vi "source_measure.vi"(8 "error in (no error)":errorcluster, 11 "Input parameters":T1={"Measurement type"=enum."Debug", "Sensor type"=enum."HPK_8in_256", "Identifier"="test.txt", "Open after execution?"=FALSE, "Plot after execution?"=FALSE, "Display channel"=0, "Voltage Delay (s)"=0.5, "Switch Delay (s)"=0.01, "VISA resource name source"="", "VISA resource name DMM"="", "VISA resource name LCR"="", "Compliance  Level (A)"=10.0, "Voltage Limit (V)"=1000.0, "Data storage location"="", "Scan voltages"="", "Use source as DMM?"=FALSE, "LCR signal frequenzy (Hz)"=10.0, "DMM device"=enum."Keithley2001", "Sampling number"=1, "Use env. sensors on"=enum."Sensirion sht1x/7x", "Switchboard Handle"=0, "Use Switchboard"=FALSE, "LCR signal voltage (V)"=10000.0, "Repeat"=1, "Scan voltages IV"="", "Scan voltages CV"="", "Hex pad numbers?"=FALSE, "Set measurement type"=enum."Debug", "Custom pad scan"="", "IV voltage Delay (s)"=0.5, "CV voltage Delay (s)"=0.5, "Needle measurement?"=FALSE, "Comments"="test.txt", "LCR signal frequenzy (kHz)"=10.0, "Compliance  Level (uA)"=10.0, "Open Correction Array"=array2304x3[6912 elements], "Current set voltage"=0.0, "Last set voltage"=0.0, "Current channel"=0, "Last OpenCorrection index"=-1, "Total curr/vltg every x steps"=10, "Current channel iteration"=0, "No CV corrections"=FALSE, "Mapfile"="", "Corrfile"="", "IV voltage file"=path "", "CV voltage file"=path "", "IV Switch Delay (s)"=0.01, "CV Switch Delay (s)"=0.01, "Invert polarity"=FALSE, "Set debug dirs"=FALSE, "Is n on p"=FALSE} {"CV Switch Delay (s)" format="%#_13g"; "IV Switch Delay (s)" format="%#_13g"; "Last set voltage" format="%#_13g"; "Current set voltage" format="%#_13g"; "CV voltage Delay (s)" format="%#_13g"; "IV voltage Delay (s)" format="%#_13g"; "Voltage Limit (V)" format="%#_13g"; "Voltage Delay (s)" format="%#_13g"; "Switch Delay (s)" format="%#_13g"}) -> (0 "error out":errorcluster, 2 "Total current":dbl, 3 "Input parameters":T1={"Measurement type"=enum."Debug", "Sensor type"=enum."HPK_8in_256", "Identifier"="test.txt", "Open after execution?"=FALSE, "Plot after execution?"=FALSE, "Display channel"=0, "Voltage Delay (s)"=0.5, "Switch Delay (s)"=0.01, "VISA resource name source"="", "VISA resource name DMM"="", "VISA resource name LCR"="", "Compliance  Level (A)"=10.0, "Voltage Limit (V)"=1000.0, "Data storage location"="", "Scan voltages"="", "Use source as DMM?"=FALSE, "LCR signal frequenzy (Hz)"=10.0, "DMM device"=enum."Keithley2001", "Sampling number"=1, "Use env. sensors on"=enum."Sensirion sht1x/7x", "Switchboard Handle"=0, "Use Switchboard"=FALSE, "LCR signal voltage (V)"=10000.0, "Repeat"=1, "Scan voltages IV"="", "Scan voltages CV"="", "Hex pad numbers?"=FALSE, "Set measurement type"=enum."Debug", "Custom pad scan"="", "IV voltage Delay (s)"=0.5, "CV voltage Delay (s)"=0.5, "Needle measurement?"=FALSE, "Comments"="test.txt", "LCR signal frequenzy (kHz)"=10.0, "Compliance  Level (uA)"=10.0, "Open Correction Array"=array2304x3[6912 elements], "Current set voltage"=0.0, "Last set voltage"=0.0, "Current channel"=0, "Last OpenCorrection index"=-1, "Total curr/vltg every x steps"=10, "Current channel iteration"=0, "No CV corrections"=FALSE, "Mapfile"="", "Corrfile"="", "IV voltage file"=path "", "CV voltage file"=path "", "IV Switch Delay (s)"=0.01, "CV Switch Delay (s)"=0.01, "Invert polarity"=FALSE, "Set debug dirs"=FALSE, "Is n on p"=FALSE} {"CV Switch Delay (s)" format="%#_13g"; "IV Switch Delay (s)" format="%#_13g"; "Last set voltage" format="%#_13g"; "Current set voltage" format="%#_13g"; "CV voltage Delay (s)" format="%#_13g"; "IV voltage Delay (s)" format="%#_13g"; "Voltage Limit (V)" format="%#_13g"; "Voltage Delay (s)" format="%#_13g"; "Switch Delay (s)" format="%#_13g"}, 4 "Compliance reached?":bool, 5 "Actual voltage":dbl)   [LabVIEW 2016]
doc: "Determines current voltage and current through source meter."
uses:
  input_params.ctl
  <instrlib>/Keithley 24XX/Keithley 24XX.lvlib
panel:
  out "Effective resistance":sgl
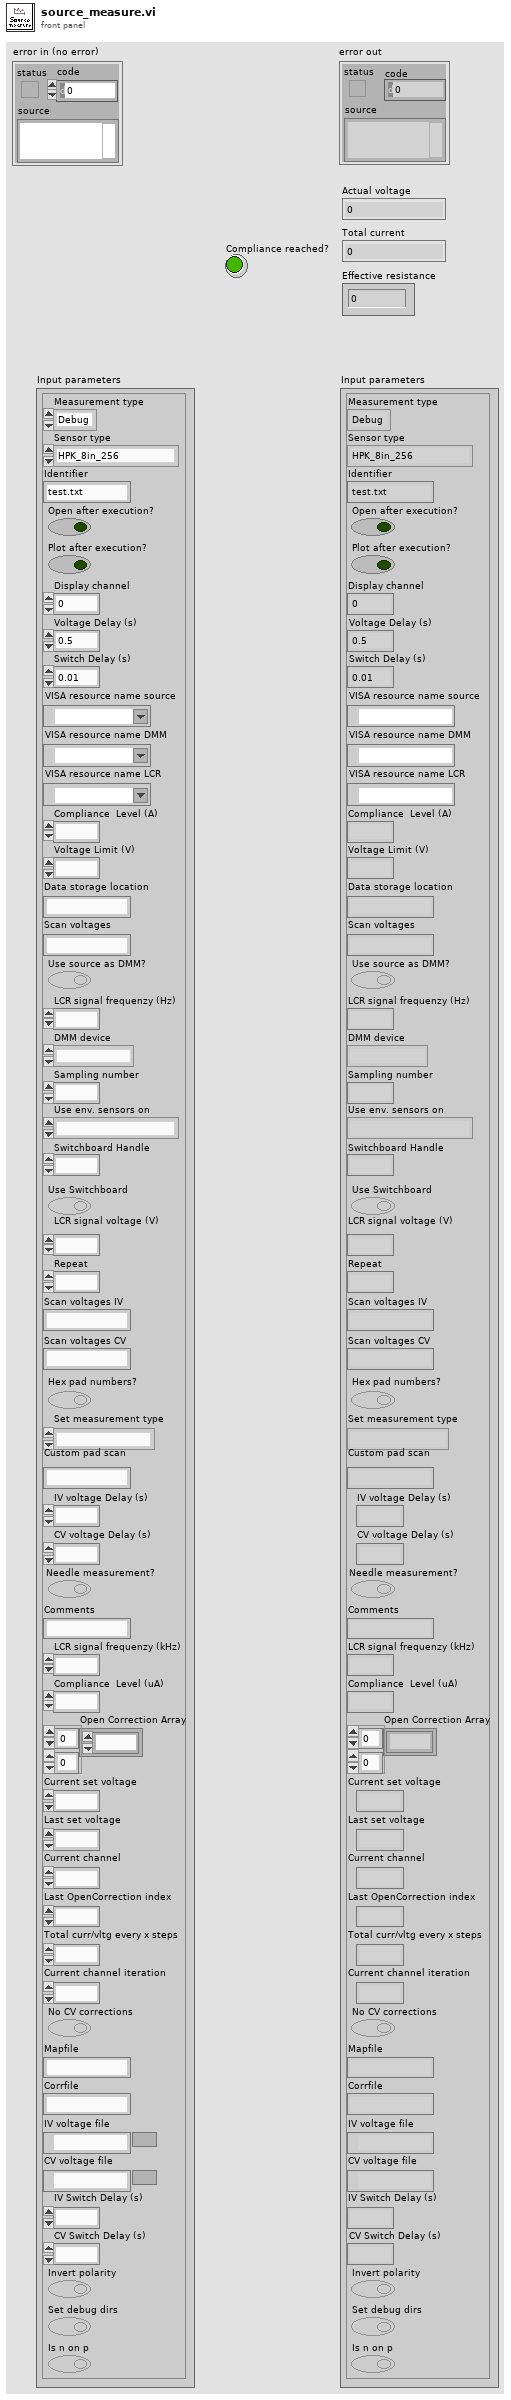
[diagram p1: front panel]
types:
  T1 = typedef "input_params.ctl" = cluster{"Measurement type":enum16{"IV", "CV", "Debug", "Test_contact"}, "Sensor type":enum16{"HPK_6in_135", "HPK_8in_256", "IFX_8in_256", "Diode", "HPK_6in_256", "Full matrix"}, "Identifier":string, "Open after execution?":bool, "Plot after execution?":bool, "Display channel":i32, "Voltage Delay (s)":dbl, "Switch Delay (s)":dbl, "VISA resource name source":refnum<visa-resource-name>, "VISA resource name DMM":refnum<visa-resource-name>, "VISA resource name LCR":refnum<visa-resource-name>, "Compliance  Level (A)":dbl, "Voltage Limit (V)":dbl, "Data storage location":string, "Scan voltages":string, "Use source as DMM?":bool, "LCR signal frequenzy (Hz)":dbl, "DMM device":enum16{"Keithley2001", "Keithley2450", "Keithley2410", "Keithley6487"}, "Sampling number":i32, "Use env. sensors on":enum16{"Sensirion sht1x/7x", "Switch Matrix", "Probecard"}, "Switchboard Handle":u32, "Use Switchboard":bool, "LCR signal voltage (V)":dbl, "Repeat":i32, "Scan voltages IV":string, "Scan voltages CV":string, "Hex pad numbers?":bool, "Set measurement type":enum16{"IV", "CV", "Debug", "Test_contact", "IV+CV"}, "Custom pad scan":string, "IV voltage Delay (s)":dbl, "CV voltage Delay (s)":dbl, "Needle measurement?":bool, "Comments":string, "LCR signal frequenzy (kHz)":dbl, "Compliance  Level (uA)":dbl, "Open Correction Array":dbl[][], "Current set voltage":dbl, "Last set voltage":dbl, "Current channel":i32, "Last OpenCorrection index":i32, "Total curr/vltg every x steps":i32, "Current channel iteration":i32, "No CV corrections":bool, "Mapfile":string, "Corrfile":string, "IV voltage file":path, "CV voltage file":path, "IV Switch Delay (s)":dbl, "CV Switch Delay (s)":dbl, "Invert polarity":bool, "Set debug dirs":bool, "Is n on p":bool}
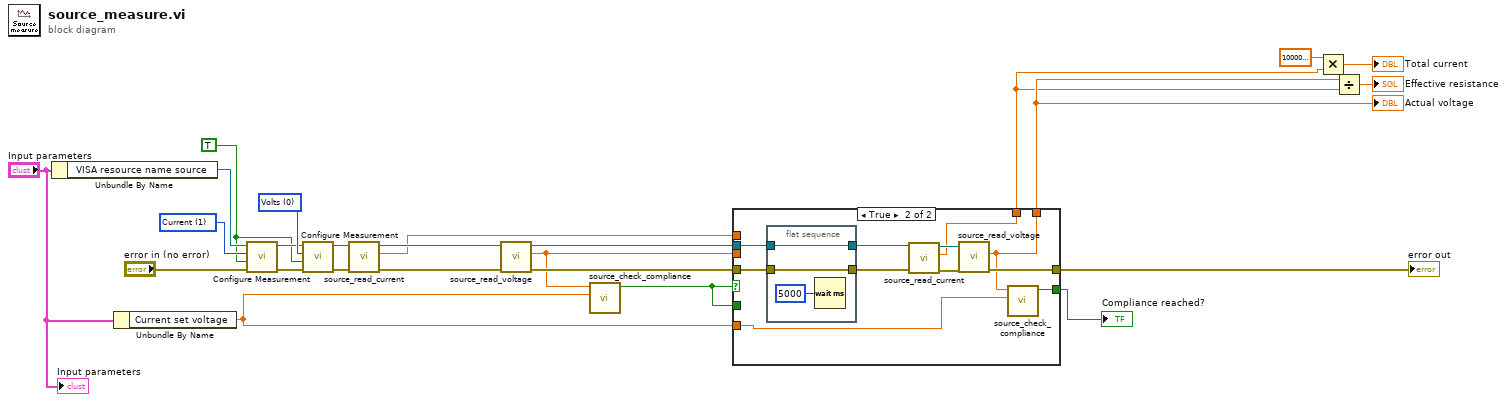
[diagram p0: block diagram]
diagram:
  w19 = TRUE
  w22 = u16 0 items=["Volts", "Current", "Resistance"] ("Function (0: Volts)")
  w23 = u16 1 items=["Volts", "Current", "Resistance"] ("Function (0: Volts)")
  n1 = Unbundle By Name("Input parameters") -> ("VISA resource name source"=w25:refnum<visa-resource-name>)
  n2 = Unbundle By Name("Input parameters") -> ("Current set voltage"=w1:dbl)
  n3 = call <instrlib>:"Configure Measurement.vi"("error in (no error)"="error in (no error)", "Enable Auto Range (T:Enable)"=w19, "Function (0: Volts)"=w23, "VISA resource name"=w25) -> ("error out"=w21:errorcluster, "VISA resource name out"=w20:refnum<visa-resource-name>)  [unwired: 6 in]
  n4 = call <instrlib>:"Configure Measurement.vi"("error in (no error)"=w21, "Enable Auto Range (T:Enable)"=w19, "Function (0: Volts)"=w22, "VISA resource name"=w20) -> ("error out"=w16:errorcluster, "VISA resource name out"=w15:refnum<visa-resource-name>)  [unwired: 6 in]
  n5 = call "source_read_current.vi"("error in (no error)"=w16, "VISA resource name"=w15) -> ("error out"=w14:errorcluster, "Value"=w5:sgl, "VISA resource name out"=w13:refnum<visa-resource-name>)  [unwired: 7 in]
  n6 = call "source_read_voltage.vi"("error in (no error)"=w14, "VISA resource name"=w13) -> ("error out"=w10:errorcluster, "Value"=w6:sgl, "VISA resource name out"=w2:refnum<visa-resource-name>)  [unwired: 7 in]
  n7 = call "source_check_compliance.vi"("Target voltage"=w1, "Actual voltage"=w6) -> ("Is compliance?"=w8:bool)  [unwired: 9 in]
  n8 = case shown="True" w8 {
    tunnel: w10 -> [w29 w36]
    tunnel: [w29 w40] -> w9
    tunnel: w8 -> [w28 _]
    tunnel: [w28 w38] -> w7
    tunnel: w6 -> [w27 _]
    tunnel: w5 -> [w26 _]
    tunnel: [w27 w35] -> w4
    tunnel: [w26 w30] -> w3
    tunnel: w2 -> [_ w37]
    tunnel: w1 -> [_ w39]
    frame False {
    }
    frame True {
      n9 = flat-sequence {
        tunnel: w37 -> [w41]
        tunnel: w36 -> [w42]
        tunnel: [w42] -> w34
        tunnel: [w41] -> w32
        frame #0 {
          n10 = Wait (ms)(milliseconds to wait=u32 5000) -> ()  [unwired: 1 out]
        }
      }
      n11 = call "source_read_current.vi"("error in (no error)"=w34, "VISA resource name"=w32) -> ("error out"=w33:errorcluster, "Value"=w30:sgl, "VISA resource name out"=w31:refnum<visa-resource-name>)  [unwired: 7 in]
      n12 = call "source_read_voltage.vi"("error in (no error)"=w33, "VISA resource name"=w31) -> ("error out"=w40:errorcluster, "Value"=w35:sgl)  [unwired: 7 in, 1 out]
      n13 = call "source_check_compliance.vi"("Target voltage"=w39, "Actual voltage"=w35) -> ("Is compliance?"=w38:bool)  [unwired: 9 in]
    }
  }
  "Actual voltage" <- w4
  "error out" <- w9
  "Compliance reached?" <- w7
  n14 = Multiply(x=sgl 1000000000.0 ("Value"), y=w3) -> (x*y=→"Total current":sgl)
  n15 = Divide(x=w4, y=w3) -> (x/y=→"Effective resistance":sgl)
  "Input parameters" <- "Input parameters"
